vi "Merc Gen Command TCP-IP VI.vi"(2 "error in (no error)":errorcluster, 3 "Command String":string="READ:SYS:CAT", 4 "IP Address":string="172.16.136.21") -> (0 "error out":errorcluster, 1 "read data":string)   [LabVIEW 2019, in "Mercury iXX.lvlib"]
uses:
  mercury/Mercury iXX.lvlib
panel:
  in  "Clear port?":bool
  in  "Command mode?":bool caption="SCPI         Legacy"
  out "return count":u32
  # "SET:DEV:MB1.T1:TEMP:LOOP:RENA:OFF"
  # "Note about SCPI command strings.\nCommand strings are made up of nouns or verbs separated by colons.\nThe verb is either READ to get a parameter value from the instrument\nor SET to write a parameter value to the instrument.\n\nThis is followed by a noun to define whetner the command is being addressed\nto the system SYS or one of the units devices DEV.  For example to read the\nsystems time the command would be:-\nREAD:SYS:TIME\n\nWhen reading from a device the unique identity (UID) must be supplied as the\nunit may contain many devices.  The UID is a construct of motherboard, MB,\nor daughter board, DB, tag, an index number 0-8, a type letter and index\nand a type (e.g. HTR forheater).  So an example UID would be:-\nMB1.T1.TEMP which represents the index 1 device of the motherboard which\nis a temperature sensor device.\nFor a heater daughter board the UID might be:-\nDB2.H1.HTR where the 2 after DB is the slot number the daughter board is in.\nTo find out what devices are in the unit send the system catalogue command:-\nREAD:SYS:CAT.\n\nFollowing the UID is the actual command.  So to read the voltage signal from\nthe motherboard temperature reading circuit device the command would be:-\nREAD:DEV:MB1.T1:TEMP:SIG:VOLT\nthe reponse should be: -\nSTAT:DEV:MB1.T1:TEMP:SIG:VOLT:11.2345mV\n\nAs an example, to set the voltage limit (VLIM) of the mother board heater output\ncircuit device to 20 volts, the command would be:-\nSET:DEV:MB0.H1:HTR:VLIM:20\nIf successful the response would be:-\nSTAT:SET:DEV:MB0.H1:HTR:VLIM:20:VALID\nIf unsuccessful a response of the form:-\nSTAT:SET:DEV:MB0.H1:HTR:VLIM:20:INVALID\nThe word INVALID will appear directly following the item in the command that the  unit doesn't understand."
  # "SET:DEV:MB1.T1:TEMP:CAL:CAL"
  # "SET:DEV:MB1.T1:TEMP:LOOP:TSET:294.9"
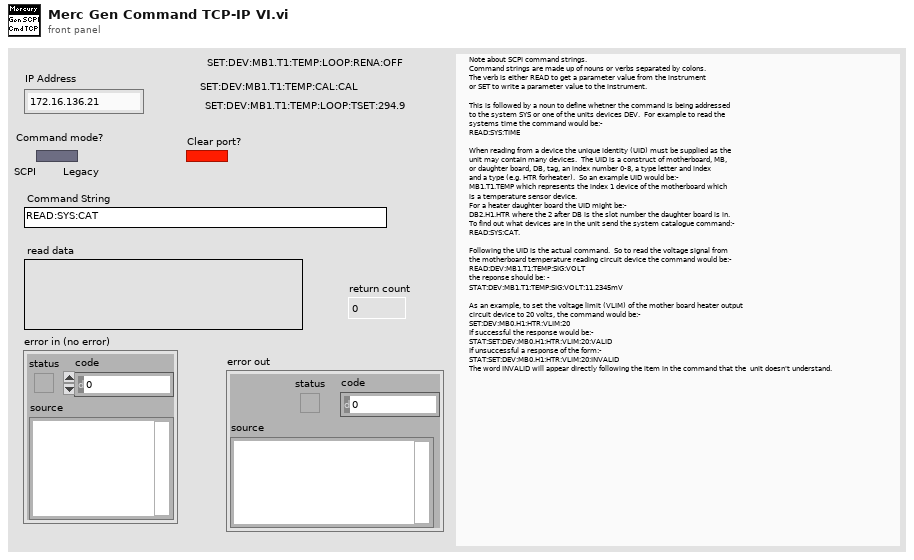
[diagram p1: front panel]
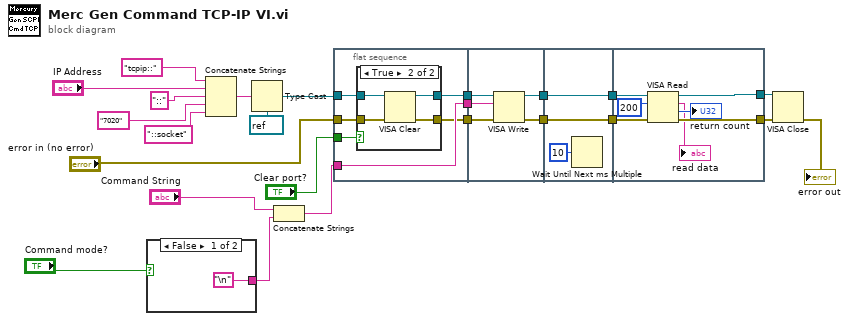
[diagram p0: block diagram]
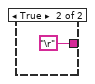
[diagram p2: hidden frame]
diagram:
  n1 = case shown="False" "Command mode?" {
    tunnel: ["\n" "\r"] -> w3
    frame False {
    }
    frame True {
    }
  }
  n2 = Concatenate Strings("tcpip::" ("string"), "IP Address", "::" ("string"), "7020" ("string"), "::socket" ("string")) -> (w14:string)
  n3 = Type Cast(type=refnum<visa-resource-name> refnum ("VISA resource name"), x=w14) -> (*(type *) &x=w7:refnum<visa-resource-name>)
  n4 = Concatenate Strings("Command String", w3) -> (w10:string)
  n5 = flat-sequence {
    tunnel: "error in (no error)" -> [w30]
    tunnel: w10 -> [w32]
    tunnel: [w31] -> w22
    tunnel: [w32] -> w21
    tunnel: [w29] -> w20
    tunnel: w7 -> [w28]
    tunnel: "Clear port?" -> [w27]
    tunnel: [w41] -> w19
    tunnel: [w40] -> w18
    tunnel: w22 -> [w43]
    tunnel: w21 -> [w42]
    tunnel: w20 -> [w39]
    tunnel: [w46] -> w17
    tunnel: w19 -> [w46]
    tunnel: w18 -> [w45]
    tunnel: [w45] -> w16
    tunnel: w17 -> [w52]
    tunnel: w16 -> [w51]
    tunnel: [w50] -> w5
    tunnel: [w49] -> w6
    frame #0 {
      n6 = case shown="True" w27 {
        tunnel: [w34 w38] -> w31
        tunnel: w30 -> [w33 w37]
        tunnel: [w33 w36] -> w29
        tunnel: w28 -> [w34 w35]
        frame False {
        }
        frame True {
          n7 = VISA Clear(VISA resource name=w35, error in (no error)=w37) -> (VISA resource name out=w38:refnum<visa-resource-name>, error out=w36:errorcluster)
        }
      }
    }
    frame #1 {
      n8 = VISA Write(VISA resource name=w43, write buffer=w42, error in (no error)=w39) -> (VISA resource name out=w41:refnum<visa-resource-name>, error out=w40:errorcluster)  [unwired: 1 out]
    }
    frame #2 {
      n9 = Wait Until Next ms Multiple(millisecond multiple=u32 10) -> ()  [unwired: 1 out]
    }
    frame #3 {
      n10 = VISA Read(VISA resource name=w52, byte count=u32 200, error in (no error)=w51) -> (VISA resource name out=w49:refnum<visa-resource-name>, read buffer=→"read data":string, return count=→"return count":u32, error out=w50:errorcluster)
    }
  }
  n11 = VISA Close(VISA resource name=w6, error in (no error)=w5) -> (error out=→"error out":errorcluster)
